vi "CRYASIOSampleRatesSupported.vi"(11 "error in (no error)":errorcluster) -> (0 "SampleRates Array Str":string[](array[string]), 1 "SampleRates Array":dbl[](array[numeric]), 3 "error out":errorcluster)   [LabVIEW 2013]
uses:
  CRY_ASIO.dll
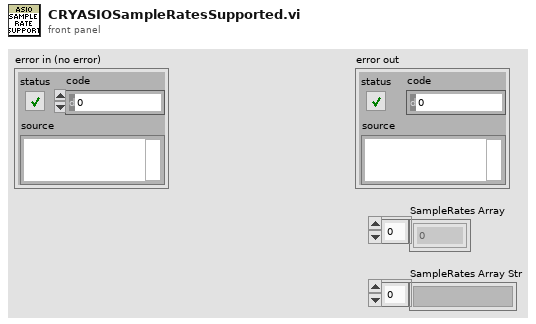
[diagram p1: front panel]
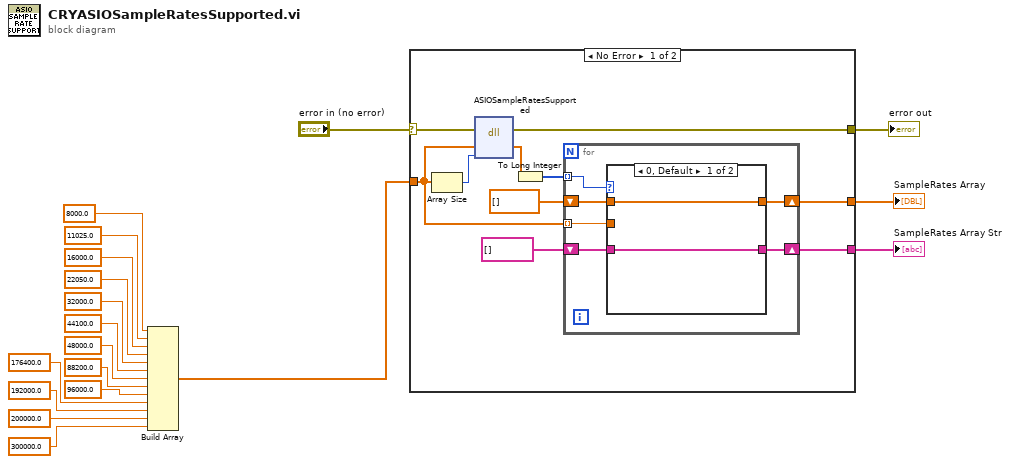
[diagram p0: block diagram]
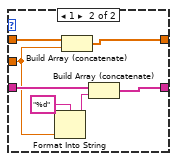
[diagram p2: hidden frame]
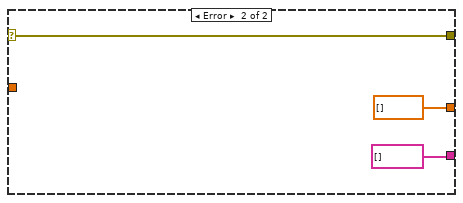
[diagram p3: hidden frame]
diagram:
  n1 = Build Array(8000.0 ("element"), 11025.0 ("element"), 16000.0 ("element"), 22050.0 ("element"), 32000.0 ("element"), 44100.0 ("element"), 48000.0 ("element"), 88200.0 ("element"), 96000.0 ("element"), 176400.0 ("element"), 192000.0 ("element"), 200000.0 ("element"), 300000.0 ("element")) -> (w3:dbl[])
  n2 = case shown="No Error" "error in (no error)" {
    selector: "error in (no error)" -> [w28 w46]
    tunnel: [w27 w46] -> w17
    tunnel: w3 -> [w24 _]
    tunnel: [w21 dbl[] [] ("SampleRate Result")] -> w2
    tunnel: [w19 string[] [] ("SampleRates Array Str")] -> w1
    frame No Error {
      n3 = Array Size(array=w24) -> (size(s)=w26:i32)
      n4 = dll-call lib="D:/LabView_Project/CRY6181/CRY_ASIO.dll" fn="ASIOSampleRatesSupported"(error in=w28, "fsArray"=w24, "count"=w26) -> (error out=w27:errorcluster, "fsArray"=w25:dbl[])  [unwired: 4 in, 1 out]
      n5 = To Long Integer(number=w25) -> (32bit integer=w22:i32[])
      n6 = for {
        tunnel: w22 -> [w34] mode=indexing
        tunnel: w24 -> [w32] mode=indexing
        shift-right: [w31] -> w21
        shift-left: dbl[] [] ("SampleRate Result") -> [w33]
        shift-right: [w29] -> w19
        shift-left: string[] [] ("SampleRates Array Str") -> [w30]
        n7 = case shown="0, Default" w34 {
          tunnel: w33 -> [w36 w43]
          tunnel: w32 -> [_ w39]
          tunnel: [w36 w42] -> w31
          tunnel: w30 -> [w35 w41]
          tunnel: [w35 w37] -> w29
          frame 0, Default {
          }
          frame 1 {
            n8 = Format Into String(format string="%d", w39) -> (resulting string=w38:string)  [unwired: 2 in, 1 out]
            n9 = Build Array (concatenate)(w43, w39) -> (w42:dbl[])
            n10 = Build Array (concatenate)(w41, w38) -> (w37:string[])
          }
        }
      }
    }
    frame Error {
    }
  }
  "error out" <- w17
  "SampleRates Array" <- w2
  "SampleRates Array Str" <- w1
